vi "DisConnect.vi"(8 "error in (no error)":errorcluster, 11 "Client In":refnum<class "Client.lvclass">) -> (0 "error out":errorcluster, 2 "ret":i32, 3 "Client out":refnum<class "Client.lvclass">)   [LabVIEW 2017, in "opcua.lvlib" / "Client.lvclass"]
uses:
  Client.lvclass
  Client.lvclass/Client.ctl
  opcua32.dll
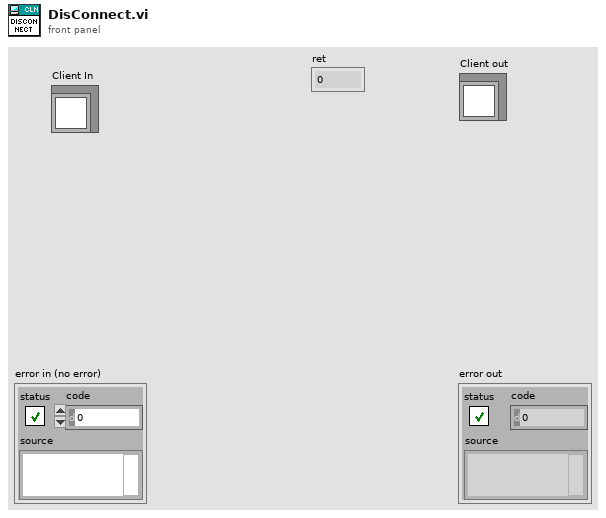
[diagram p1: front panel]
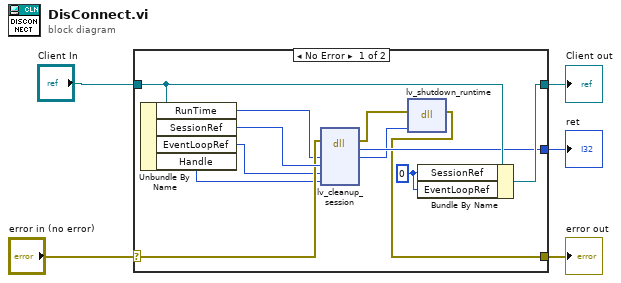
[diagram p0: block diagram]
diagram:
  n1 = case shown="No Error" "error in (no error)" {
    selector: "error in (no error)" -> [w14 w18]
    tunnel: [w8 w18] -> w4
    tunnel: [w17 w19] -> w3
    tunnel: "Client In" -> [w16 w19]
    tunnel: [w13 _] -> w1
    frame No Error {
      w11 = u64 0 ("SessionRef")
      n2 = Unbundle By Name(w16) -> ("RunTime"=w10:u64, "SessionRef"=w15:u64, "EventLoopRef"=w12:u64, "Handle"=w6:u64)
      n3 = dll-call lib="C:/Users/Andrey/Desktop/opcua-labview/opcua-lvlib/opcua*.dll" fn="lv_cleanup_session"(error in=w14, "RunTime"=w10, "session"=w15, "event_loop"=w12, "handle_in"=w6) -> (error out=w9:errorcluster, "return type"=w13:i32, "RunTime"=w7:u64)  [unwired: 5 in, 1 out]
      n4 = dll-call lib="C:/Users/Andrey/Desktop/opcua-labview/opcua-lvlib/opcua*.dll" fn="lv_shutdown_runtime"(error in=w9, "RunTime"=w7) -> (error out=w8:errorcluster)  [unwired: 4 in, 1 out]
      n5 = Bundle By Name(cluster=w16, "SessionRef"=w11, "EventLoopRef"=w11) -> (w17:refnum<class "Client.lvclass">)
    }
    frame Error {
    }
  }
  "error out" <- w4
  "Client out" <- w3
  "ret" <- w1
